vi "FGV_Error Handler.vi"(7 "Current Account":i32, 8 "error in (no error)":errorcluster, 9 "Clear Error?":bool, 10 "Classification":T1, 11 "Command":T2) -> (0 "error out":errorcluster, 2 "System Error":bool, 3 "Session Error":bool)   [LabVIEW 2012]
uses:
  DataType/FGV_Error Handler_Command.ctl
  DataType/FGV_Error Handler_Classification.ctl
  DataType/FGV_Error Handler_Error log.ctl
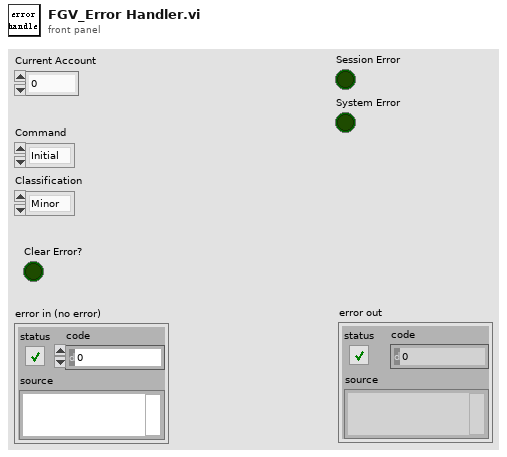
[diagram p1: front panel]
types:
  T1 = typedef "FGV_Error Handler_Classification.ctl" = enum16{"Minor", "Session", "System"}
  T2 = typedef "FGV_Error Handler_Command.ctl" = enum16{"Initial", "Handle", "Check", "Close", "Set Account"}
  T3 = typedef "FGV_Error Handler_Error log.ctl" = cluster{timestamp, "Classification":T1, "Current Account":i32, "error in (no error)":errorcluster}
  T4 = enum16{"open", "replace", "create", "open or create", "replace or create", "replace or create with confirmation"}
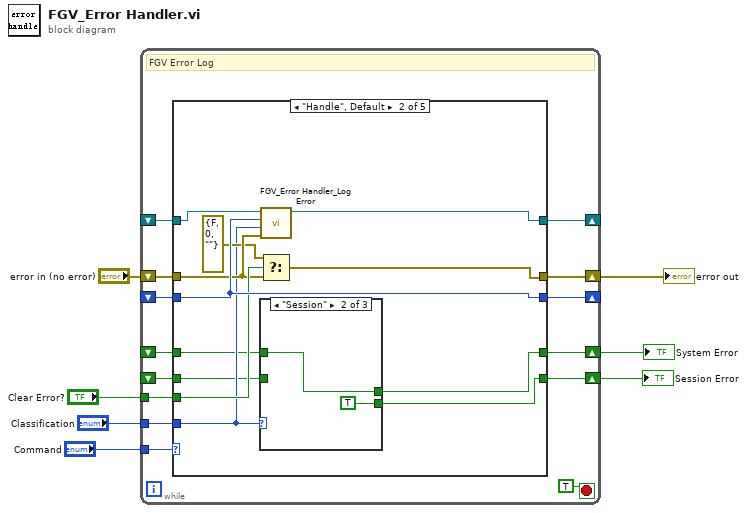
[diagram p0: block diagram]
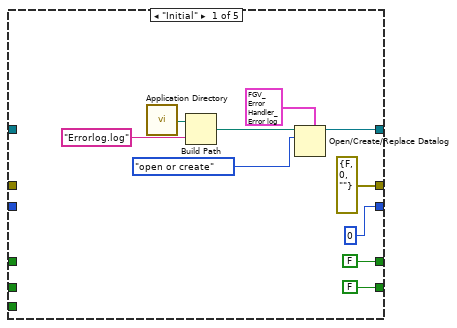
[diagram p2: hidden frame]
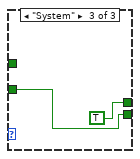
[diagram p4: hidden frame]
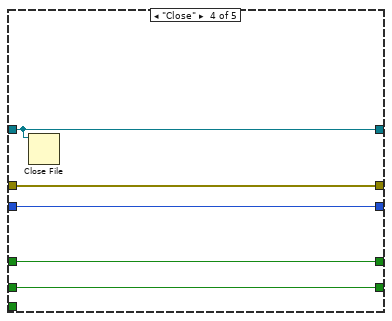
[diagram p6: hidden frame]
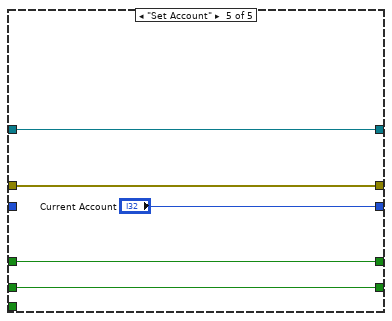
[diagram p7: hidden frame]
diagram:
  n1 = while {
    tunnel: "Command" -> [w21]
    tunnel: "Clear Error?" -> [w17]
    tunnel: "Classification" -> [w15]
    shift-right: [w14] -> w2
    shift-left: _ -> [w12]
    shift-right: [w13] -> w1
    shift-left: _ -> [w11]
    shift-right: [w9] -> _
    shift-left: _ -> [w16]
    shift-right: [w10] -> _
    shift-left: _ -> [w8]
    shift-right: [w20] -> w6
    shift-left: "error in (no error)" -> [w19]
    stop <- TRUE stop-if-true
    # "FGV Error Log"
    n2 = case shown="\"Handle\", Default" w21 {
      tunnel: [errorcluster {"status"=FALSE, "code"=0, "source"=""} ("error in (no error)") w40 w51 w59 w62] -> w20
      tunnel: w19 -> [_ w38 w51 w59 w62]
      tunnel: w17 -> [_ w39 _ _ _]
      tunnel: w16 -> [_ w41 w52 w56 _]
      tunnel: w15 -> [_ w36 _ _ _]
      tunnel: [FALSE ("Session Error") w35 w54 w57 w60] -> w14
      tunnel: [FALSE ("System Error") w33 w53 w58 w61] -> w13
      tunnel: w12 -> [_ w34 w54 w57 w60]
      tunnel: w11 -> [_ w32 w53 w58 w61]
      tunnel: [w28 w43 w50 w55 w63] -> w10
      tunnel: [0 ("Current Account") w41 w52 w56 "Current Account"] -> w9
      tunnel: w8 -> [_ w42 w50 w55 w63]
      frame "Initial" {
        n3 = call <vilib>:"Application Directory.vi"() -> ("Application Directory"=w26:path)
        n4 = Build Path(base path=w26, name or relative path="Errorlog.log") -> (appended path=w25:path)
        n5 = Open/Create/Replace Datalog(5:T3 {timestamp(0 s since 1904-01-01), "Classification"=enum."Minor", "Current Account"=0, "error in (no error)"={"status"=FALSE, "code"=0, "source"=""}}, 10:T4."open or create" ("operation (0:open)"), 11:w25) -> (3:w28:refnum<k1>)  [unwired: 3 in, 2 out]
      }
      frame "Handle", Default {
        n6 = case shown="\"Session\"" w36 {
          tunnel: [w45 TRUE ("Session Error") w49] -> w35
          tunnel: w34 -> [w45 _ w49]
          tunnel: [w44 w46 TRUE ("System Error")] -> w33
          tunnel: w32 -> [w44 w46 _]
          frame "Minor", Default {
          }
          frame "Session" {
          }
          frame "System" {
          }
        }
        n7 = call "FGV_Error Handler_Log Error.vi"("error in (no error)"=w38, "Classification"=w36, "Current Account"=w41, "Refnum in"=w42) -> ("Refnum out"=w43:refnum<k1>)  [unwired: 7 in]
        n8 = Select(t=errorcluster {"status"=FALSE, "code"=0, "source"=""}, s=w39, f=w38) -> (s? t:f=w40:errorcluster)
      }
      frame "Check" {
      }
      frame "Close" {
        n9 = Close File(refnum=w55) -> ()  [unwired: 1 in, 2 out]
      }
      frame "Set Account" {
      }
    }
  }
  "error out" <- w6
  "Session Error" <- w2
  "System Error" <- w1
